vi "Teleop.vi"(10 "Match Info":T1={"Autonomous Elapsed Seconds"=0.0, "TeleOp Elapsed Seconds"=0.0, "Disabled Elapsed Seconds"=0.0, "Visited Autonomous"=FALSE, "Visited TeleOp"=FALSE, "Visited Disabled"=FALSE, "Autonomous Settings"={"Autonomous Style"=enum."Independent", "VI Refnum"=refnum}}, 11 "Call Context":T2) -> ()   [LabVIEW 2018]
doc: "This VI is called for each enabled TeleOp packet received from the DS. It is typically used to read from joysticks and other inputs and update I/O or setpoints for timed control loops. It should complete and return within 20 milliseconds or risk missing DS packets."
uses:
  <vilib>/Rock Robotics/WPI/DriverStation/WPI_DriverStationDerivedRobotMode.ctl
  <vilib>/Rock Robotics/WPI/DriverStation/WPI_DriverStationMatch Info.ctl
  Support Code/Joystick Vals.ctl
  Elevator/Implementation/Infrastructure/Positions.ctl
  <vilib>/Rock Robotics/WPI/Utilities/WPI_GetSetVariantRefNum.vi
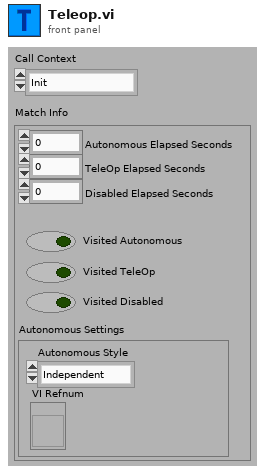
[diagram p1: front panel]
types:
  T1 = typedef "WPI_DriverStationMatch Info.ctl" = cluster{"Autonomous Elapsed Seconds":dbl, "TeleOp Elapsed Seconds":dbl, "Disabled Elapsed Seconds":dbl, "Visited Autonomous":bool, "Visited TeleOp":bool, "Visited Disabled":bool, "Autonomous Settings":cluster{"Autonomous Style":enum16{"Iterative", "Independent"}, "VI Refnum":refnum<vi>}}
  T2 = typedef "WPI_DriverStationDerivedRobotMode.ctl" = enum16{"Init", "Execute", "Stop"}
  T3 = typedef "Joystick Vals.ctl" = cluster{"Driver Axes":dbl[], "Co-Driver Axes":dbl[], "Driver Buttons":bool[], "Co-Driver Buttons":bool[], "Driver POV":i16[], "Co-Driver POV":i16[], "Climb Buttons":bool[], "Climb Axes":dbl[]}
  T4 = typedef "WPI_JoystickDevRef.ctl" = cluster{"Device":T5}
  T5 = typedef "WPI_JoystickDeviceEnum.ctl" = enum16{"USB 0", "USB 1", "USB 2", "USB 3", "USB 4", "USB 5"}
  T6 = typedef "Positions.ctl" = enum16{"MANUAL", "Bottom Pannel", "Bottom Cargo", "Feeder Station", "Cargo Ship Cargo", "Middle Pannel", "Middle Cargo", "Top Pannel", "Top Cargo"}
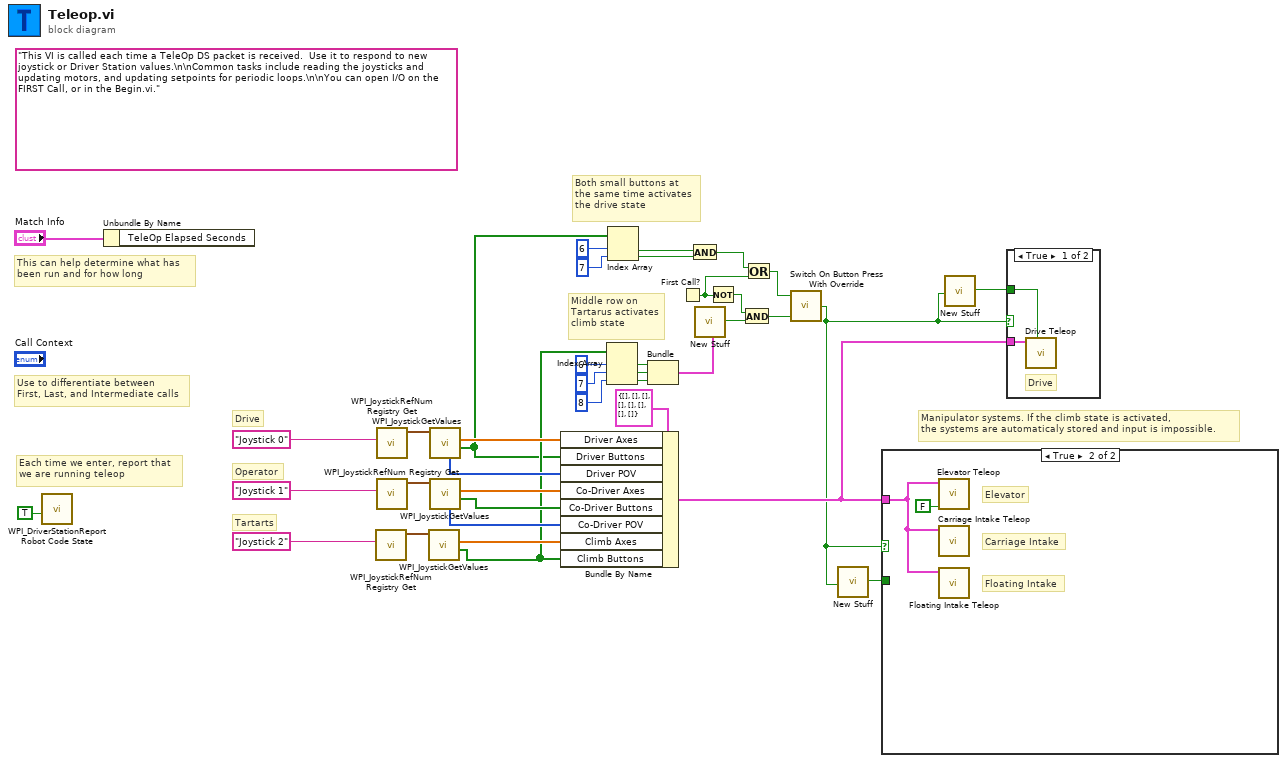
[diagram p0: block diagram]
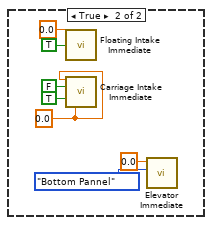
[diagram p3: hidden frame]
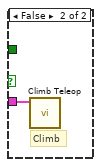
[diagram p4: hidden frame]
diagram:
  (unwired) "This VI is called each time a TeleOp DS packet is received.  Use it to respond to new joystick or Driver Station values.\n\nCommon tasks include reading the joysticks and updating motors, and updating setpoints for periodic loops.\n\nYou can open I/O on the FIRST Call, or in the Begin.vi."
  # "Manipulator systems. If the climb state is activated,\nthe systems are automaticaly stored and input is impossible."
  # "Middle row on\nTartarus activates\nclimb state"
  # "Both small buttons at\nthe same time activates\nthe drive state"
  # "Tartarts"
  # "Operator"
  # "Drive"
  # "Each time we enter, report that\nwe are running teleop"
  # "Use to differentiate between\nFirst, Last, and Intermediate calls"
  # "This can help determine what has\nbeen run and for how long"
  n1 = call <vilib>:"WPI_DriverStationReport Robot Code State.vi"("TeleOp"=TRUE ("Autonomous")) -> ()  [unwired: 10 in, 1 out]
  n2 = Unbundle By Name("Match Info") -> ()  [unwired: 1 out]
  n3 = call <vilib>:"WPI_JoystickRefNum Registry Get.vi"("refnum name"="Joystick 2") -> ("JoystickDevRef"=w25:T4)  [unwired: 1 in, 9 out]
  n4 = call <vilib>:"WPI_JoystickRefNum Registry Get.vi"("refnum name"="Joystick 0") -> ("JoystickDevRef"=w35:T4)  [unwired: 1 in, 9 out]
  n5 = call <vilib>:"WPI_JoystickRefNum Registry Get.vi"("refnum name"="Joystick 1") -> ("JoystickDevRef"=w34:T4)  [unwired: 1 in, 9 out]
  n6 = call <vilib>:"WPI_JoystickGetValues.vi"("JoystickDevRef"=w25) -> ("Buttons"=w23:bool[], "Axes"=w24:dbl[])  [unwired: 6 in, 3 out]
  n7 = call <vilib>:"WPI_JoystickGetValues.vi"("JoystickDevRef"=w35) -> ("Buttons"=w1:bool[], "Axes"=w29:dbl[], "POVs"=w30:i16[])  [unwired: 6 in, 2 out]
  n8 = call <vilib>:"WPI_JoystickGetValues.vi"("JoystickDevRef"=w34) -> ("Buttons"=w27:bool[], "Axes"=w28:dbl[], "POVs"=w32:i16[])  [unwired: 6 in, 2 out]
  n9 = Bundle By Name(cluster=T3 {"Driver Axes"=[], "Co-Driver Axes"=[], "Driver Buttons"=[], "Co-Driver Buttons"=[], "Driver POV"=[], "Co-Driver POV"=[], "Climb Buttons"=[], "Climb Axes"=[]} ("Cluster"), "Driver Axes"=w29, "Driver Buttons"=w1, "Driver POV"=w30, "Co-Driver Axes"=w28, "Co-Driver Buttons"=w27, "Co-Driver POV"=w32, "Climb Axes"=w24, "Climb Buttons"=w23) -> (w4:T3)
  n10 = Index Array(array=w23, index #1=6 ("index"), index #2=7 ("index"), index #3=8 ("index")) -> (element #1=w19:bool, element #2=w18:bool, element #3=w17:bool)
  n11 = Index Array(array=w1, index #1=6 ("index"), index #2=7 ("index")) -> (element #1=w13:bool, element #2=w12:bool)
  n12 = Bundle(w19, w18, w17) -> (w16:cluster{bool, bool, bool})  [unwired: 1 in]
  n13 = First Call?() -> (First Call?: T/F=w7:bool)
  n14 = And(x=w13, y=w12) -> (x .and. y?=w8:bool)
  n15 = call "New Stuff.vi"("Variant 9"=w16) -> ("x != y?"=w10:bool)  [unwired: 26 in]
  n16 = Not(x=w7) -> (.not. x?=w11:bool)
  n17 = And(x=w11, y=w10) -> (x .and. y?=w9:bool)
  n18 = Or(x=w8, y=w7) -> (x .or. y?=w6:bool)
  n19 = call "Switch On Button Press With Override.vi"("Override False"=w9, "Override True"=w6) -> ("Output"=w3:bool)  [unwired: 1 in]
  n20 = call "New Stuff.vi"("Variant 16"=w3) -> ("x != y?"=w5:bool)  [unwired: 26 in]
  n21 = case shown="True" w3 {
    tunnel: w4 -> [_ w47]
    tunnel: w5 -> [w39 _]
    frame False {
      n22 = case shown="False" w39 {
        frame False {
        }
        frame True {
          w42 = 0.0 ("Setpoint")
          n23 = call "Floating Intake Immediate.vi"("Setpoint"=0.0, "Retract"=TRUE) -> ()  [unwired: 13 in, 1 out]
          n24 = call "Carriage Intake Immediate.vi"("Setpoint Left"=w42, "Extend"=FALSE, "Close"=TRUE, "Setpoint Right"=w42) -> ()  [unwired: 11 in, 1 out]
          n25 = call "Elevator Immediate.vi"("Position"=Positions."Bottom Pannel", "Setpoint"=0.0) -> ()  [unwired: 9 in, 1 out]
        }
      }
    }
    frame True {
      # "Elevator"
      # "Floating Intake"
      # "Carriage Intake"
      n26 = call "Elevator Teleop.vi"("Disabled"=FALSE, "Cluster"=w47) -> ()  [unwired: 10 in]
      n27 = call "Carriage Intake Teleop.vi"("Cluster"=w47) -> ()  [unwired: 11 in]
      n28 = call "Floating Intake Teleop.vi"("Cluster"=w47) -> ()  [unwired: 11 in]
    }
  }
  n29 = call "New Stuff.vi"("Variant 16"=w3) -> ("x != y?"=w2:bool)  [unwired: 26 in]
  n30 = case shown="True" w3 {
    tunnel: w4 -> [w50 w51]
    tunnel: w2 -> [w49 _]
    frame True {
      # "Drive"
      n31 = call "Drive Teleop.vi"("New Stuff"=w49, "Cluster"=w50) -> ()  [unwired: 10 in]
    }
    frame False {
      # "Climb"
      n32 = call "Climb Teleop.vi"("Cluster"=w51) -> ()  [unwired: 11 in]
    }
  }
